vi "MR.vi"(0 "Motion Resource In":refnum<k21>) -> (1 "Motion Resource Out":refnum<k21>, 2 "number":u32 format="%x")   [LabVIEW 2010]
panel:
  out "xml string":string
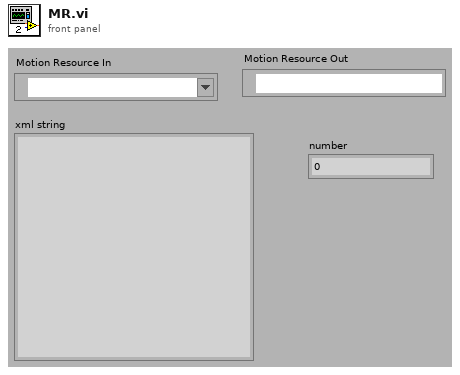
[diagram p1: front panel]
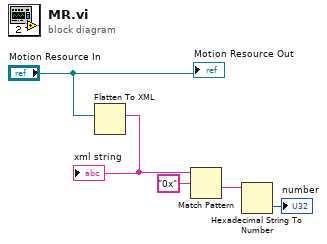
[diagram p0: block diagram]
diagram:
  n1 = Flatten To XML(anything="Motion Resource In") -> (xml string=w4:string)
  "xml string" <- w4
  n2 = Match Pattern(string=w4, regular expression="0x") -> (after substring=w2:string)  [unwired: 4 out]
  n3 = Hexadecimal String To Number(string=w2) -> (number=→"number":u32)  [unwired: 3 out]
  "Motion Resource Out" <- "Motion Resource In"
